vi "store2ADCToFileAverage.vi"(2 "Xtalk on":bool, 4 "S.Dev.":dbl[](array[numeric]), 5 "Write to disk":T1(ring), 6 "Averages":dbl[](array[numeric]), 7 "iterationXtalk":u32, 8 "keithleyVoltage":dbl, 9 "attenuateVal":u16) -> (0 "error out":errorcluster)   [LabVIEW 2014]
uses:
  <vilib>/Analysis/baseanly.llb/Mean (DBL).vi
  Global 1.vi
  <vilib>/Analysis/NI_AALBase.lvlib
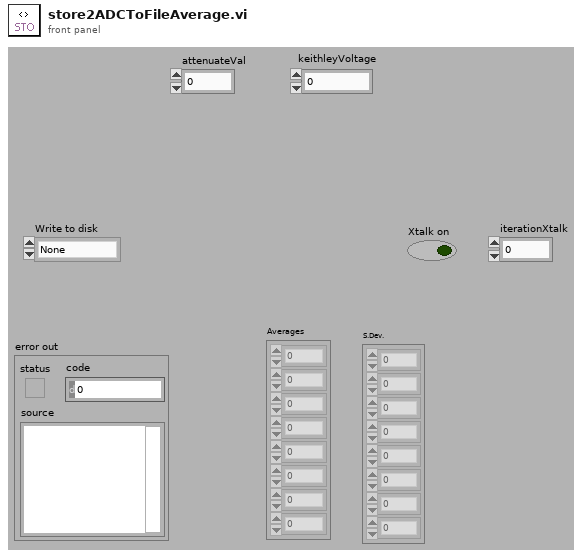
[diagram p1: front panel]
types:
  T1 = enum16{"None", "Average", "StdDev", "AvgStdDev", "ChanAverage", "All"}
  T2 = enum16{"open", "replace", "create", "open or create", "replace or create", "replace or create with confirmation"}
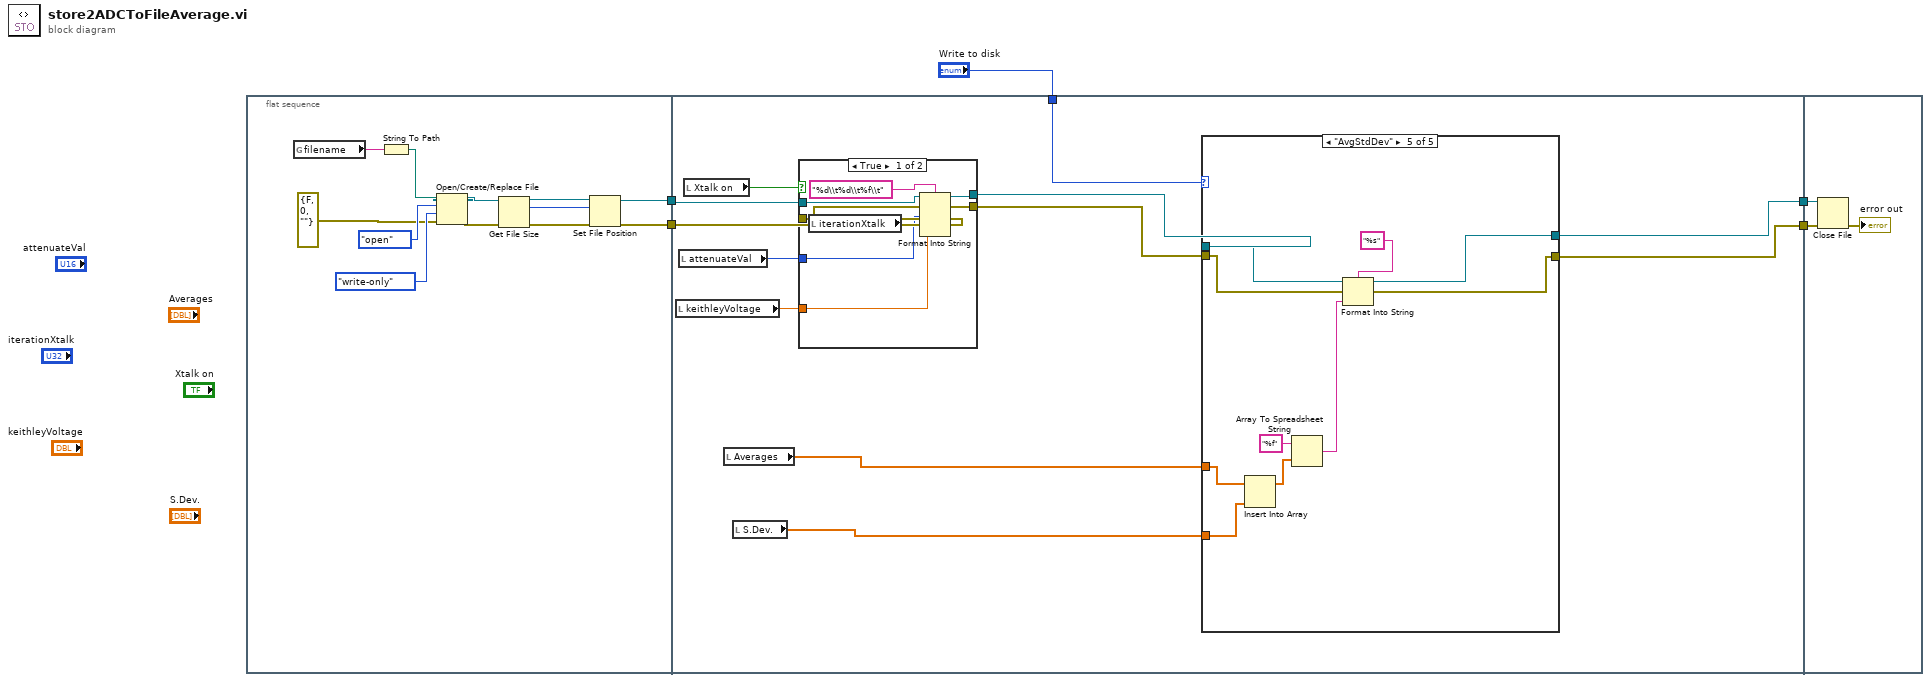
[diagram p0: block diagram]
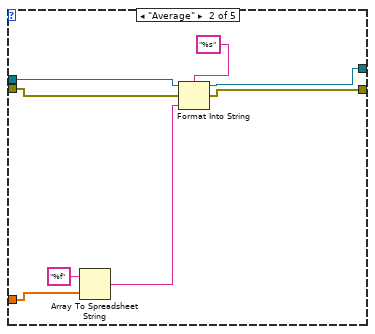
[diagram p3: hidden frame]
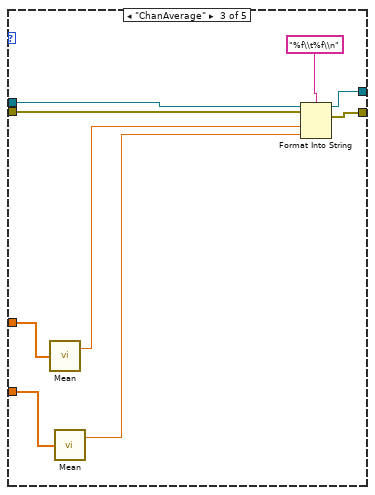
[diagram p4: hidden frame]
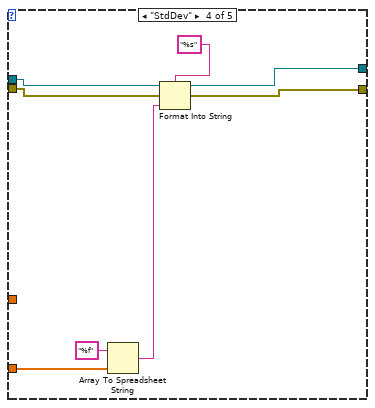
[diagram p5: hidden frame]
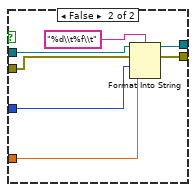
[diagram p6: hidden frame]
diagram:
  n1 = flat-sequence {
    tunnel: [w8] -> w5
    tunnel: [w7] -> w4
    tunnel: w5 -> [w28]
    tunnel: w4 -> [w29]
    tunnel: [w27] -> w3
    tunnel: [w26] -> w2
    tunnel: "Write to disk" -> [w22]
    tunnel: w3 -> [w84]
    tunnel: w2 -> [w82]
    frame #0 {
      n2 = global read "Global 1.vi" "filename"() -> (w6:string)
      n3 = String To Path(string=w6) -> (path=w15:path)
      n4 = Open/Create/Replace File(file path (use dialog)=w15, error in=errorcluster {"status"=FALSE, "code"=0, "source"=""} ("error out"), operation (0:open)=T2."open", access (0:read/write)=enum16{"read/write", "read-only", "write-only"}."write-only") -> (refnum out=w12:refnum<file>, error out=w11:errorcluster)  [unwired: 3 out]
      n5 = Get File Size(file=w12, error in=w11) -> (refnum out=w9:refnum<file>, size (in bytes)=w17:i64, 0:w10:errorcluster)
      n6 = Set File Position(offset (in bytes) (0)=w17, refnum=w9, error in=w10) -> (refnum out=w8:refnum<file>, error out=w7:errorcluster)  [unwired: 1 out]
    }
    frame #1 {
      n7 = local read "keithleyVoltage"() -> (w20:dbl)
      n8 = local read "attenuateVal"() -> (w21:u16)
      n9 = local read "Xtalk on"() -> (w25:bool)
      n10 = local read "Averages"() -> (w19:dbl[])
      n11 = local read "S.Dev."() -> (w18:dbl[])
      n12 = case shown="True" w25 {
        tunnel: w28 -> [w73 w80]
        tunnel: w29 -> [w72 w79]
        tunnel: [w71 w78] -> w24
        tunnel: [w70 w77] -> w23
        tunnel: w21 -> [w68 w76]
        tunnel: w20 -> [w67 w75]
        frame True {
          n13 = local read "iterationXtalk"() -> (w69:u32)
          n14 = Format Into String(format string="%d\\t%d\\t%f\\t", initial string=w73, error in=w72, w69, w68, w67) -> (resulting string=w71:refnum<file>, error out=w70:errorcluster)
        }
        frame False {
          n15 = Format Into String(format string="%d\\t%f\\t", initial string=w80, error in=w79, w76, w75) -> (resulting string=w78:refnum<file>, error out=w77:errorcluster)
        }
      }
      n16 = case shown="\"AvgStdDev\"" w22 {
        tunnel: [w31 w35 w48 w53 w63] -> w27
        tunnel: [w30 w36 w47 w52 w62] -> w26
        tunnel: w24 -> [w31 w38 w45 w55 w65]
        tunnel: w23 -> [w30 w37 w44 w54 w64]
        tunnel: w19 -> [_ w33 w41 _ w60]
        tunnel: w18 -> [_ _ w40 w50 w59]
        frame "None", Default {
        }
        frame "Average" {
          n17 = Array To Spreadsheet String(array=w33, 3:"%f" ("format string")) -> (spreadsheet string=w32:string)  [unwired: 1 out]
          n18 = Format Into String(format string="%s", initial string=w38, error in=w37, w32) -> (resulting string=w35:refnum<file>, error out=w36:errorcluster)
        }
        frame "ChanAverage" {
          n19 = call-poly <vilib>:"Mean.vi"("X"=w41) -> ("mean"=w43:dbl)  [unwired: 1 out]
          n20 = call-poly <vilib>:"Mean.vi"("X"=w40) -> ("mean"=w42:dbl)  [unwired: 1 out]
          n21 = Format Into String(format string="%f\\t%f\\n", initial string=w45, error in=w44, w43, w42) -> (resulting string=w48:refnum<file>, error out=w47:errorcluster)
        }
        frame "StdDev" {
          n22 = Array To Spreadsheet String(array=w50, 3:"%f" ("format string")) -> (spreadsheet string=w49:string)  [unwired: 1 out]
          n23 = Format Into String(format string="%s", initial string=w55, error in=w54, w49) -> (resulting string=w53:refnum<file>, error out=w52:errorcluster)
        }
        frame "AvgStdDev" {
          n24 = Insert Into Array(array=w60, new element=w59) -> (w58:dbl[])  [unwired: 1 in]
          n25 = Array To Spreadsheet String(array=w58, 3:"%f" ("format string")) -> (spreadsheet string=w57:string)  [unwired: 1 out]
          n26 = Format Into String(format string="%s", initial string=w65, error in=w64, w57) -> (resulting string=w63:refnum<file>, error out=w62:errorcluster)
        }
      }
    }
    frame #2 {
      n27 = Close File(refnum=w84, error in=w82) -> (error out=→"error out":errorcluster)  [unwired: 1 out]
    }
  }
